vi "Process each line scan.vi"() -> ()   [LabVIEW 2012]
uses:
  <vilib>/Analysis/3filter.llb/Filter Passband Type.ctl
  <vilib>/Analysis/NI_AALBase.lvlib
panel:
  in  "filter type":T1
  in  "High Cutoff Freq":dbl=300.0
  in  "Offset Diff":dbl=2.0
  in  "Offset Normal":dbl=2.0
  out "Differential data":dbl[][](graph)
  out "Normal data":dbl[][](graph)
  in  "Low Cutoff Freq":dbl=50.0
  in  "Open":bool
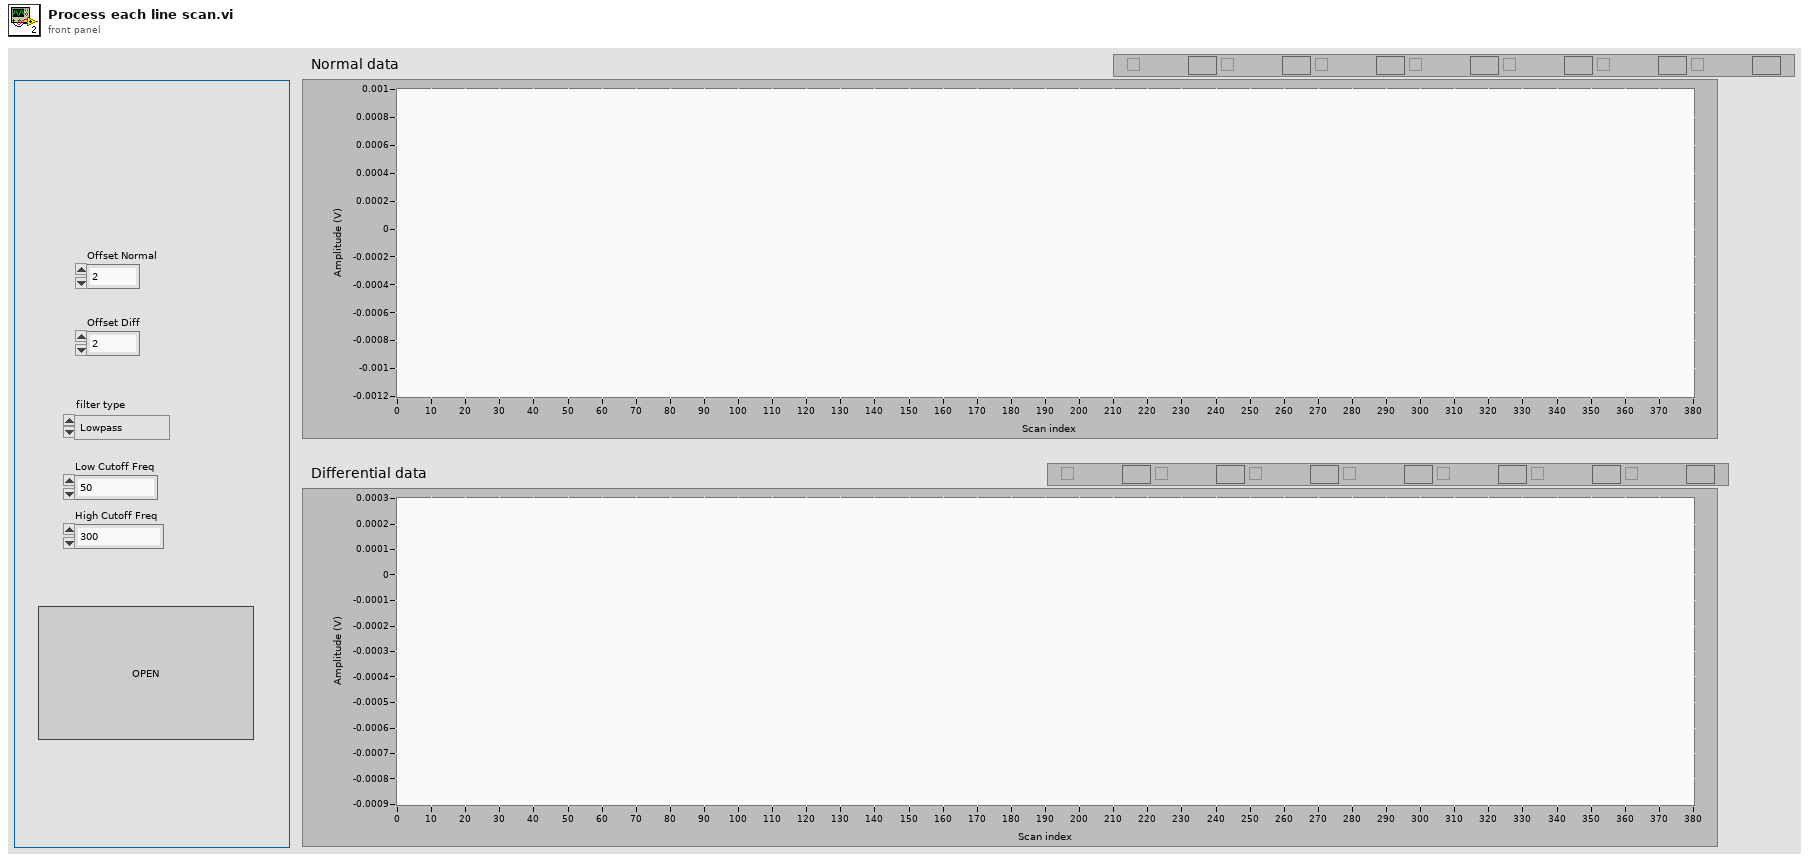
[diagram p1: front panel]
types:
  T1 = typedef "NI_AALBase.lvlib/Filter Passband Type.ctl" = enum32{"Lowpass", "Highpass", "Bandpass", "Bandstop"}
  T2 = typedef "NI_Matrix.lvlib/RealMatrix.ctl" = dbl[][]
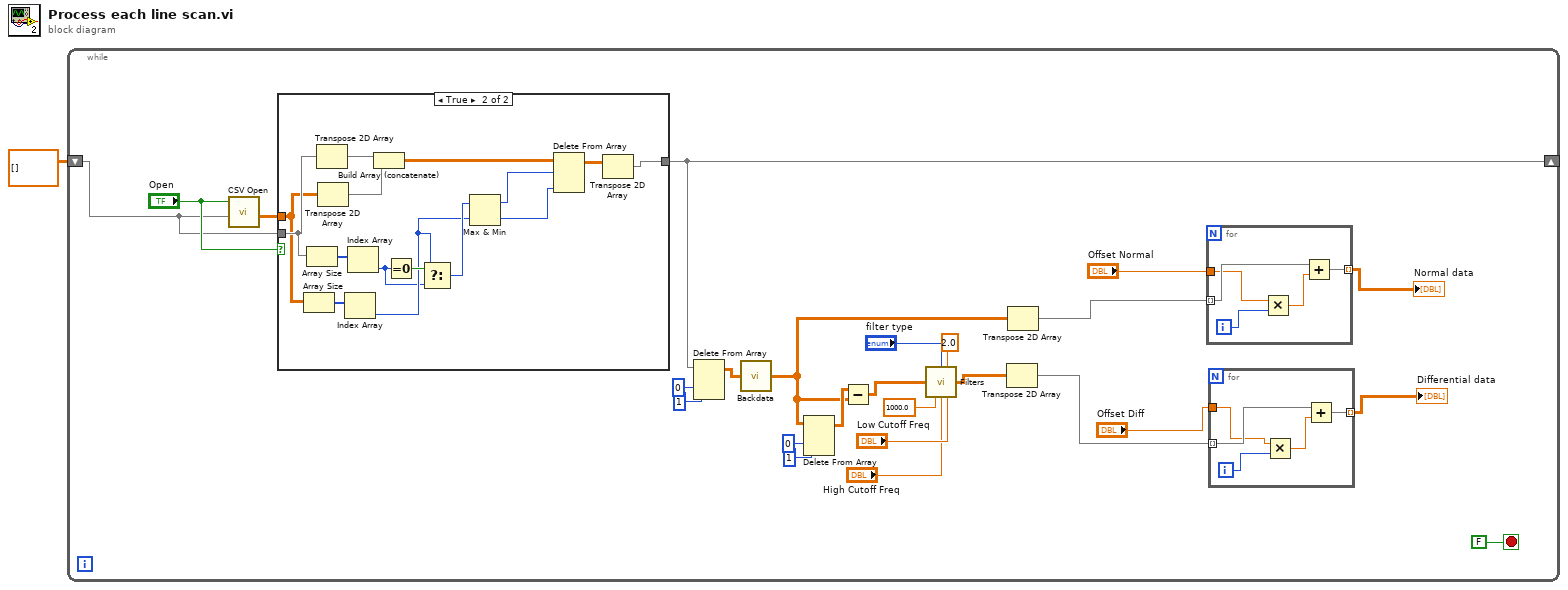
[diagram p0: block diagram]
diagram:
  n1 = while {
    shift-right: [w7] -> _
    shift-left: dbl[][] [] ("2D Array Out") -> [w15]
    stop <- FALSE stop-if-true
    n2 = call "CSV Open.vi"("2D Array In"=w15, "Open"="Open") -> ("2D Array Out"=w16:dbl[][])  [unwired: 9 in]
    n3 = case shown="True" "Open" {
      tunnel: [w37 w44] -> w7
      tunnel: w16 -> [w37 w47]
      tunnel: w15 -> [_ w50]
      frame False {
      }
      frame True {
        n4 = Array Size(array=w47) -> (size(s)=w48:i32[])
        n5 = Array Size(array=w50) -> (size(s)=w49:i32[])
        n6 = Transpose 2D Array(2D array=w50) -> (transposed array=w52:dbl[][])
        n7 = Transpose 2D Array(2D array=w47) -> (transposed array=w51:dbl[][])
        n8 = Index Array(array=w48) -> (element=w39:i32)  [unwired: 1 in]
        n9 = Index Array(array=w49) -> (element=w38:i32)  [unwired: 1 in]
        n10 = Build Array (concatenate)(w52, w51) -> (w46:dbl[][])
        n11 = Equal To 0?(x=w38) -> (x = 0?=w41:bool)
        n12 = Select(t=w39, s=w41, f=w38) -> (s? t:f=w40:i32)
        n13 = Max & Min(x=w40, y=w39) -> (max(x,y)=w43:i32, min(x,y)=w42:i32)
        n14 = Delete From Array(array=w46, length=w43, index (col)=w42) -> (array with subset deleted=w45:dbl[][])  [unwired: 1 in, 1 out]
        n15 = Transpose 2D Array(2D array=w45) -> (transposed array=w44:dbl[][])
      }
    }
    n16 = Delete From Array(array=w7, length=1 ("길이"), index (row)=0 ("인덱스 (행)")) -> (array with subset deleted=w6:dbl[][])  [unwired: 1 in, 1 out]
    n17 = call "Backdata.vi"("Array in"=w6) -> ("Array out"=w5:dbl[][])  [unwired: 2 in]
    n18 = Delete From Array(array=w5, length=1 ("길이"), index (row)=0 ("인덱스 (행)")) -> (array with subset deleted=w22:dbl[][])  [unwired: 1 in, 1 out]
    n19 = Subtract ("Subtract.vi")(x=w22, y=w5) -> (x-y=w2:dbl[][])
    n20 = call "Filters.vi"("filter type"="filter type", "Order"=2.0, "Input data"=w2, "Sampling Freq"=1000.0, "High Cutoff Freq"="High Cutoff Freq", "Low Cutoff Freq"="Low Cutoff Freq") -> ("Filterd Data Matrix"=w26:T2)  [unwired: 9 in]
    n21 = Transpose 2D Array(2D array=w26) -> (transposed array=w4:T2)
    n22 = Transpose 2D Array(2D array=w5) -> (transposed array=w12:dbl[][])
    n23 = for {
      tunnel: "Offset Normal" -> [w32]
      tunnel: w12 -> [w33] mode=indexing
      tunnel: [w34] -> w3 mode=indexing
      i -> [w36]
      n24 = Multiply(x=w32, y=w36) -> (x*y=w35:dbl)
      n25 = Add(x=w33, y=w35) -> (x+y=w34:dbl[])
    }
    "Normal data" <- w3
    n26 = for {
      tunnel: "Offset Diff" -> [w27]
      tunnel: w4 -> [w28] mode=indexing
      tunnel: [w29] -> w10 mode=indexing
      i -> [w31]
      n27 = Multiply(x=w27, y=w31) -> (x*y=w30:dbl)
      n28 = Add(x=w28, y=w30) -> (x+y=w29:dbl[])
    }
    "Differential data" <- w10
  }
